vi "Simulate Mouse Click at Position .vi"(8 "error in (no error)":errorcluster, 9 "delay between down & up (ms)":u32=100, 10 "Right-click?":bool, 11 "Mouse Position":cluster{"Horizontal":i32, "Vertical":i32}) -> (0 "error out":errorcluster)   [LabVIEW 2020]
uses:
  user32.dll
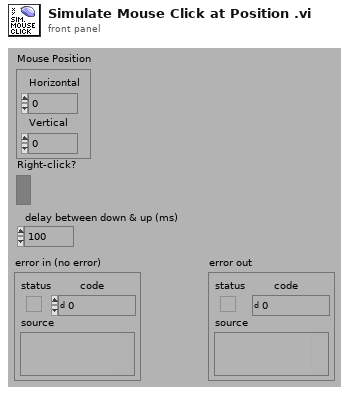
[diagram p1: front panel]
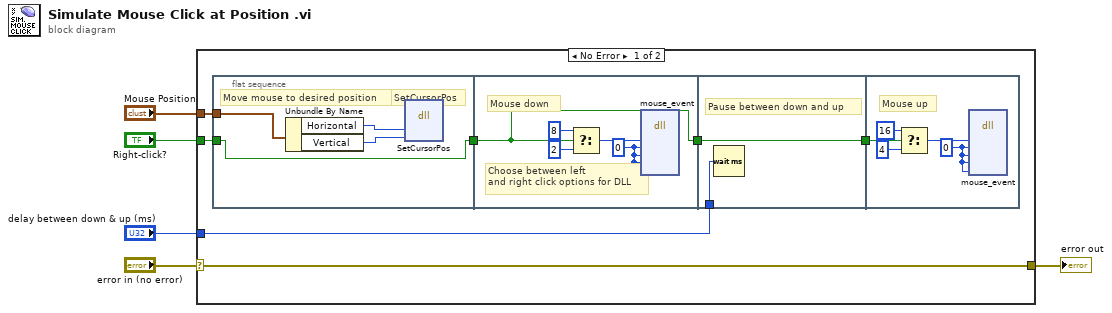
[diagram p0: block diagram]
diagram:
  n1 = case shown="No Error" "error in (no error)" {
    selector: "error in (no error)" -> [w6 w29]
    tunnel: "Right-click?" -> [w9 _]
    tunnel: "Mouse Position" -> [w8 _]
    tunnel: "delay between down & up (ms)" -> [w7 _]
    tunnel: [w6 w29] -> w2
    frame No Error {
      n2 = flat-sequence {
        tunnel: w9 -> [w13]
        tunnel: [w13] -> w12
        tunnel: w8 -> [w14]
        tunnel: w12 -> [w21]
        tunnel: [w21] -> w11
        tunnel: w11 -> [w23]
        tunnel: [w23] -> w10
        tunnel: w7 -> [w22]
        tunnel: w10 -> [w28]
        frame #0 {
          # "SetCursorPos"
          # "Move mouse to desired position"
          n3 = Unbundle By Name(w14) -> ("Horizontal"=w16:i32, "Vertical"=w15:i32)
          n4 = dll-call lib="user32.dll" fn="SetCursorPos"(w16, w15) -> ()  [unwired: 6 in, 2 out]
        }
        frame #1 {
          w17 = 0 ("dx")
          # "Choose between left\nand right click options for DLL"
          # "Mouse down"
          n5 = Select(t=u32 8, s=w21, f=u32 2) -> (s? t:f=w20:u32)
          n6 = dll-call lib="user32.dll" fn="mouse_event"("dwFlags"=w20, "dx"=w17, "dy"=w17, "dwData"=w17, "dwExtraInfo"=w17) -> ()  [unwired: 9 in, 2 out]
        }
        frame #2 {
          # "Pause between down and up"
          n7 = Wait (ms)(milliseconds to wait=w22) -> ()  [unwired: 1 out]
        }
        frame #3 {
          w24 = 0 ("dx")
          # "Mouse up"
          n8 = Select(t=u32 16, s=w28, f=u32 4) -> (s? t:f=w27:u32)
          n9 = dll-call lib="user32.dll" fn="mouse_event"("dwFlags"=w27, "dx"=w24, "dy"=w24, "dwData"=w24, "dwExtraInfo"=w24) -> ()  [unwired: 9 in, 2 out]
        }
      }
    }
    frame Error {
    }
  }
  "error out" <- w2
